vi "i2c clock fgv.vi"(7 "Function (R)":T1, 8 "error in (no error)":errorcluster caption="에러 입력(에러 없음)", 11 "i2c clock in":u8(ring) items=["400k"=3, "1M"=0, "2M"=1, "3M"=2]) -> (0 "error out":errorcluster caption="에러 출력", 3 "i2c clock out":u8(ring) items=["400k"=3, "1M"=0, "2M"=1, "3M"=2])   [LabVIEW 2020, in "Script Line_i2c.lvclass"]
uses:
  Script Line_i2c.lvclass
  Controls/(Ctrl)i2c clock fgv enum.ctl
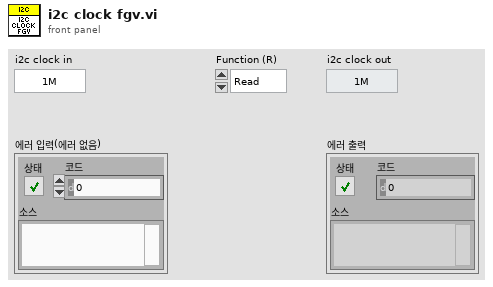
[diagram p1: front panel]
types:
  T1 = typedef "Script Line_i2c.lvclass/(Ctrl)i2c clock fgv enum.ctl" = enum16{"Read", "Write"}
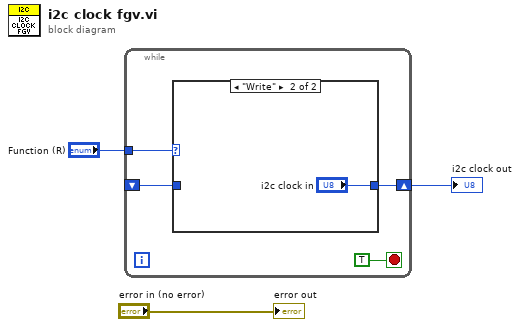
[diagram p0: block diagram]
diagram:
  n1 = while {
    tunnel: "Function (R)" -> [w6]
    shift-right: [w5] -> w1
    shift-left: _ -> [w4]
    stop <- TRUE stop-if-true
    n2 = case shown="\"Write\"" w6 {
      tunnel: [w8 "i2c clock in"] -> w5
      tunnel: w4 -> [w8 _]
      frame "Read", Default {
      }
      frame "Write" {
      }
    }
  }
  "i2c clock out" <- w1
  "error out" <- "error in (no error)"
